vi "Select indexed values.vi"(2 "Cluster":T1={"Mode"=enum."Interpolate", "Index"=[]}, 3 "Values":dbl[](array[numeric])) -> (1 "Values Out":dbl[](array[numeric]))   [LabVIEW 2022 SP3]
uses:
  Controls/Resample mode.ctl
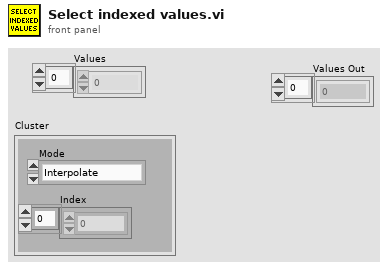
[diagram p1: front panel]
types:
  T1 = typedef "Resample mode.ctl" = cluster{"Mode":enum16{"Index", "Interpolate"}, "Index":dbl[]}
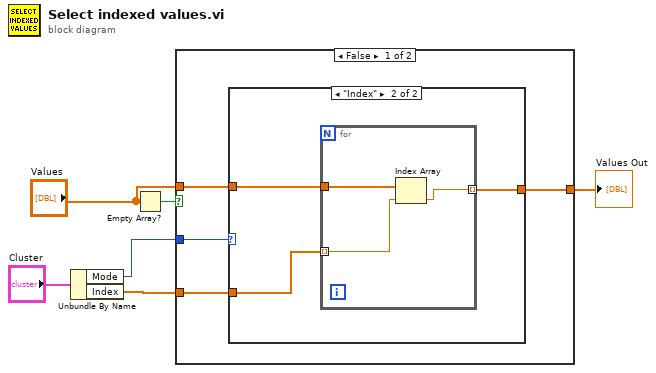
[diagram p0: block diagram]
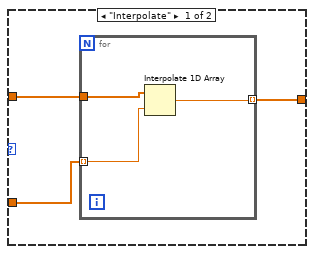
[diagram p2: hidden frame]
diagram:
  n1 = Unbundle By Name("Cluster") -> ("Mode"=w2:enum16{"Index", "Interpolate"}, "Index"=w1:dbl[])
  n2 = Empty Array?(array="Values") -> (empty?=w6:bool)
  n3 = case shown="False" w6 {
    tunnel: "Values" -> [w10 w23]
    tunnel: [w9 w23] -> w4
    tunnel: w2 -> [w8 _]
    tunnel: w1 -> [w7 _]
    frame False {
      n4 = case shown="\"Index\"" w8 {
        tunnel: w10 -> [w13 w19]
        tunnel: [w12 w18] -> w9
        tunnel: w7 -> [w11 w17]
        frame "Interpolate" {
          n5 = for {
            tunnel: w11 -> [w15] mode=indexing
            tunnel: w13 -> [w16]
            tunnel: [w14] -> w12 mode=indexing
            n6 = Interpolate 1D Array(1:w15, 2:w16) -> (0:w14:dbl)
          }
        }
        frame "Index" {
          n7 = for {
            tunnel: w17 -> [w22] mode=indexing
            tunnel: w19 -> [w21]
            tunnel: [w20] -> w18 mode=indexing
            n8 = Index Array(array=w21, index=w22) -> (element=w20:dbl)
          }
        }
      }
    }
    frame True {
    }
  }
  "Values Out" <- w4
